vi "Query Multi Eval Meas Modulation Limit Check Results.vi"(0 "VISA resource name":refnum<visa-resource-name>, 5 "Instance (1)":i32=1, 7 "Result Type (Current)":i32(ring) items=["Current"=0, "Average"=1, "Standard Deviation"=3, "Maximum"=4], 11 "error in (no error)":errorcluster) -> (4 "VISA resource name out":refnum<visa-resource-name>, 6 "Reliability":i32, 8 "Out Of Tolerance":i32, 10 "Limit Check Results":dbl[](array[numeric]), 15 "error out":errorcluster)   [LabVIEW 2015, in "Rohde&Schwarz CMP LR WPAN Measurement.lvlib"]
doc: "Returns the limit check single value results.\n\nAttribute:\n-\n\nRemote-control commands:\nCALCulate:WPAN:MEAS<i>:MEValuation:MODulation[:OFFSet]:CURRent?\nCALCulate:WPAN:MEAS<i>:MEValuation:MODulation[:OFFSet]:AVERage?\nCALCulate:WPAN:MEAS<i>:MEValuation:MODulation[:OFFSet]:SDEViation?\nCALCulate:WPAN:MEAS<i>:MEValuation:MODulation[:OFFSet]:MAXimum?"
uses:
  <instrlib>/Rohde&Schwarz CMP LR WPAN Measurement/Rohde&Schwarz CMP LR WPAN Measurement.lvlib
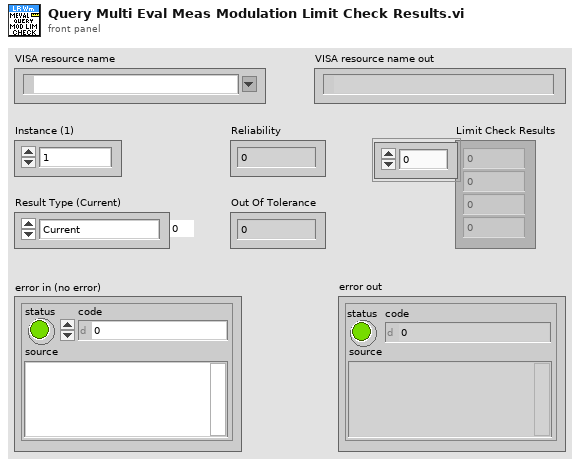
[diagram p1: front panel]
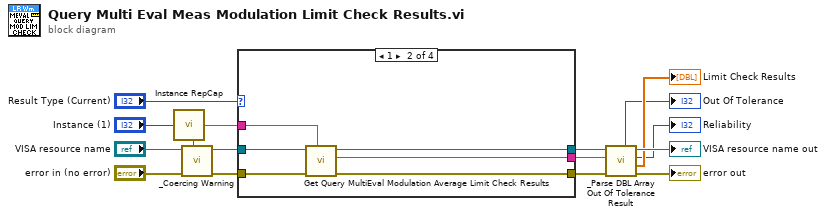
[diagram p0: block diagram]
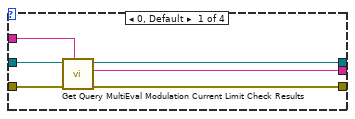
[diagram p2: hidden frame]
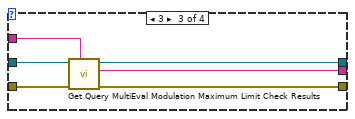
[diagram p3: hidden frame]
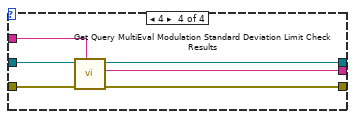
[diagram p4: hidden frame]
diagram:
  n1 = call <instrlib>:"Instance RepCap.vi"("Instance In"="Instance (1)") -> ("In Range?"=w15:bool, "RepCap Identifier Out"=w16:string)  [unwired: 1 in]
  n2 = call <instrlib>:"_Coercing Warning.vi"("In Range?"=w15, "error in (no error)"="error in (no error)", "VISA resource name"="VISA resource name") -> ("error out"=w11:errorcluster, "VISA resource name out"=w10:refnum<visa-resource-name>)  [unwired: 7 in]
  n3 = case shown="1" "Result Type (Current)" {
    tunnel: w16 -> [w22 w28 w34 w40]
    tunnel: w10 -> [w21 w27 w33 w38]
    tunnel: w11 -> [w20 w26 w32 w39]
    tunnel: [w17 w23 w29 w35] -> w5
    tunnel: [w19 w25 w31 w37] -> w4
    tunnel: [w18 w24 w30 w36] -> w3
    frame 0, Default {
      n4 = call "Get Query MultiEval Modulation Current Limit Check Results"("Repeated Capabilities"=w22, "error in (no error)"=w20, "instrument handle"=w21) -> ("error out"=w19:errorcluster, "Query MultiEval Modulation Current Limit Check Results"=w18:string, "instrument handle out"=w17:refnum<visa-resource-name>)  [unwired: 6 in]
    }
    frame 1 {
      n5 = call "Get Query MultiEval Modulation Average Limit Check Results"("Repeated Capabilities"=w28, "error in (no error)"=w26, "instrument handle"=w27) -> ("error out"=w25:errorcluster, "Query MultiEval Modulation Average Limit Check Results"=w24:string, "instrument handle out"=w23:refnum<visa-resource-name>)  [unwired: 6 in]
    }
    frame 3 {
      n6 = call "Get Query MultiEval Modulation Maximum Limit Check Results"("Repeated Capabilities"=w34, "error in (no error)"=w32, "instrument handle"=w33) -> ("error out"=w31:errorcluster, "Query MultiEval Modulation Maximum Limit Check Results"=w30:string, "instrument handle out"=w29:refnum<visa-resource-name>)  [unwired: 6 in]
    }
    frame 4 {
      n7 = call "Get Query MultiEval Modulation Standard Deviation Limit Check Results"("Repeated Capabilities"=w40, "error in (no error)"=w39, "instrument handle"=w38) -> ("error out"=w37:errorcluster, "Query MultiEval Modulation Standard Deviation Limit Check Results"=w36:string, "instrument handle out"=w35:refnum<visa-resource-name>)  [unwired: 6 in]
    }
  }
  n8 = call <instrlib>:"_Parse DBL Array Out Of Tolerance Result.vi"("error in (no error)"=w4, "Input String"=w3, "VISA resource name"=w5) -> ("error out"=→"error out":errorcluster, "Results"=→"Limit Check Results":dbl[], "Reliability"=→"Reliability":i32, "VISA resource name out"=→"VISA resource name out":refnum<visa-resource-name>, "Out Of Tolerance"=→"Out Of Tolerance":i32)  [unwired: 4 in]
